vi "Div-Cur.vi"(0 "I_S":dbl, 1 "R2":dbl, 2 "R1":dbl) -> (3 "I_EQ * R_EQ":dbl, 4 "R_EQ":dbl, 5 "I2":dbl, 6 "I1":dbl)   [LabVIEW 2010]
doc: "Calculate current at individual parallel resistors (R1, R2) within a containing circuit, provided current (I_S) of the containing circuit\n\nIn = I_s * ( R_EQ / Rn)"
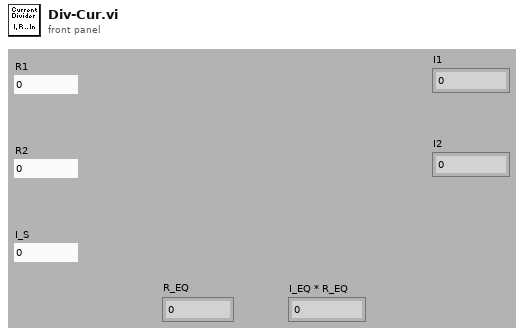
[diagram p1: front panel]
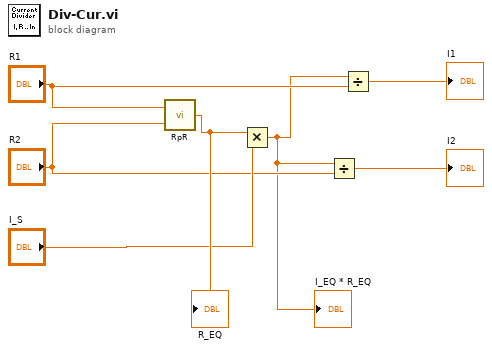
[diagram p0: block diagram]
diagram:
  n1 = call "RpR.vi"("R2"="R2", "R1"="R1") -> ("R1 // R2"=w7:dbl)  [unwired: 2 out]
  "R_EQ" <- w7
  n2 = Multiply(x=w7, y="I_S") -> (x*y=w1:dbl)
  "I_EQ * R_EQ" <- w1
  n3 = Divide(x=w1, y="R2") -> (x/y=→"I2":dbl)
  n4 = Divide(x=w1, y="R1") -> (x/y=→"I1":dbl)
